vi "HandleStop.vi"(8 "error in (no error)":errorcluster, 11 "Acquisition in":refnum<class "Acquisition.lvclass">) -> (0 "error out":errorcluster, 2 "stop?":bool, 3 "Acquisition out":refnum<class "Acquisition.lvclass">)   [LabVIEW 2018, in "Acquisition.lvclass"]
uses:
  Acquisition.lvclass
  C:/Users/observer/Desktop/Sparc4GUI/SPARC4_GUI/Server/Server.lvclass
  Server/Server.lvclass/Server.ctl
  Acquisition.lvclass/Acquisition.ctl
  Channel/Channel.lvclass
  Server/Server.lvclass
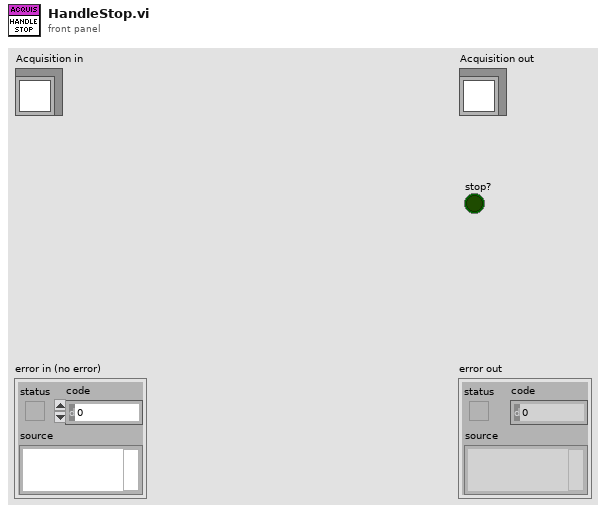
[diagram p1: front panel]
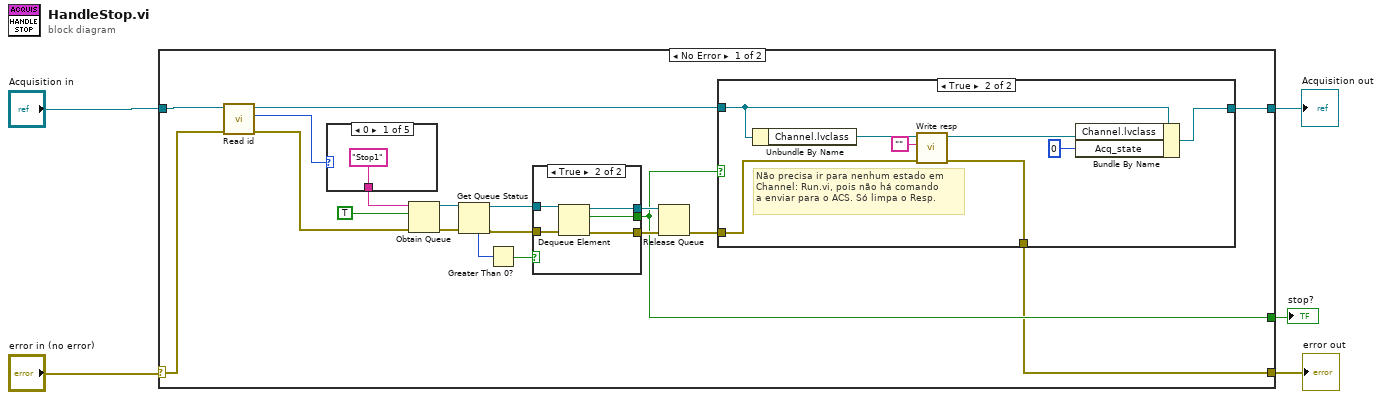
[diagram p0: block diagram]
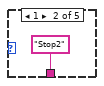
[diagram p2: hidden frame]
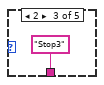
[diagram p3: hidden frame]
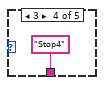
[diagram p4: hidden frame]
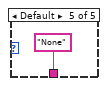
[diagram p5: hidden frame]
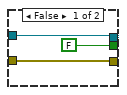
[diagram p7: hidden frame]
diagram:
  n1 = case shown="No Error" "error in (no error)" {
    selector: "error in (no error)" -> [w7 w49]
    tunnel: [w8 w49] -> w3
    tunnel: [w24 w48] -> w2
    tunnel: "Acquisition in" -> [w23 w48]
    tunnel: [w11 _] -> w1
    frame No Error {
      n2 = call "Read id.vi"("error in (no error)"=w7, "Server in"=w23) -> ("error out"=w6:errorcluster, "id"=w10:u32, "Server out"=w22:refnum<class "Acquisition.lvclass">)  [unwired: 7 in]
      n3 = case shown="0" w10 {
        tunnel: ["Stop1" ("name (unnamed)") "Stop2" ("name (unnamed)") "Stop3" ("name (unnamed)") "Stop4" ("name (unnamed)") "None" ("name (unnamed)")] -> w21
        frame 0 {
        }
        frame 1 {
        }
        frame 2 {
        }
        frame 3 {
        }
        frame Default {
        }
      }
      n4 = Obtain Queue(name (unnamed)=w21, element data type=TRUE, error in (no error)=w6) -> (queue out=w18:refnum<queue>, error out=w19:errorcluster)  [unwired: 2 in, 1 out]
      n5 = Get Queue Status(queue=w18, error in (no error)=w19) -> (queue out=w15:refnum<queue>, error out=w14:errorcluster, # elements in queue=w17:i32)  [unwired: 1 in, 5 out]
      n6 = Greater Than 0?(x=w17) -> (x > 0?=w16:bool)
      n7 = case shown="True" w16 {
        tunnel: w15 -> [w41 w46]
        tunnel: w14 -> [w40 w47]
        tunnel: [FALSE w45] -> w11
        tunnel: [w41 w44] -> w13
        tunnel: [w40 w43] -> w12
        frame False {
        }
        frame True {
          n8 = Dequeue Element(queue=w46, error in (no error)=w47) -> (queue out=w44:refnum<queue>, element=w45:bool, error out=w43:errorcluster)  [unwired: 1 in, 1 out]
        }
      }
      n9 = Release Queue(queue=w13, error in (no error)=w12) -> (error out=w9:errorcluster)  [unwired: 1 in, 2 out]
      n10 = case shown="True" w11 {
        tunnel: [w31 w38] -> w24
        tunnel: w22 -> [w31 w37]
        tunnel: w9 -> [w30 w33]
        tunnel: [w30 w32] -> w8
        frame False {
        }
        frame True {
          # "Não precisa ir para nenhum estado em \nChannel: Run.vi, pois não há comando \na enviar para o ACS. Só limpa o Resp."
          n11 = Unbundle By Name(w37) -> ("Channel.lvclass"=w36:refnum<class "Channel.lvclass">)
          n12 = call-dynamic "Write resp.vi"("error in (no error)"=w33, "resp"="", "Device in"=w36) -> ("error out"=w32:errorcluster, "Device out"=w35:refnum<class "Channel.lvclass">)  [unwired: 7 in]
          n13 = Bundle By Name(cluster=w37, "Channel.lvclass"=w35, "Acq_state"=u32 0) -> (w38:refnum<class "Acquisition.lvclass">)
        }
      }
    }
    frame Error {
    }
  }
  "error out" <- w3
  "Acquisition out" <- w2
  "stop?" <- w1
